vi "3x3 Smoothing.vi"(7 "Enable":bool, 11 "Image":u32[][](array[numeric])) -> (3 "Smoothed":u32[][](array[numeric]))   [LabVIEW 2017]
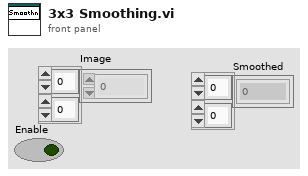
[diagram p1: front panel]
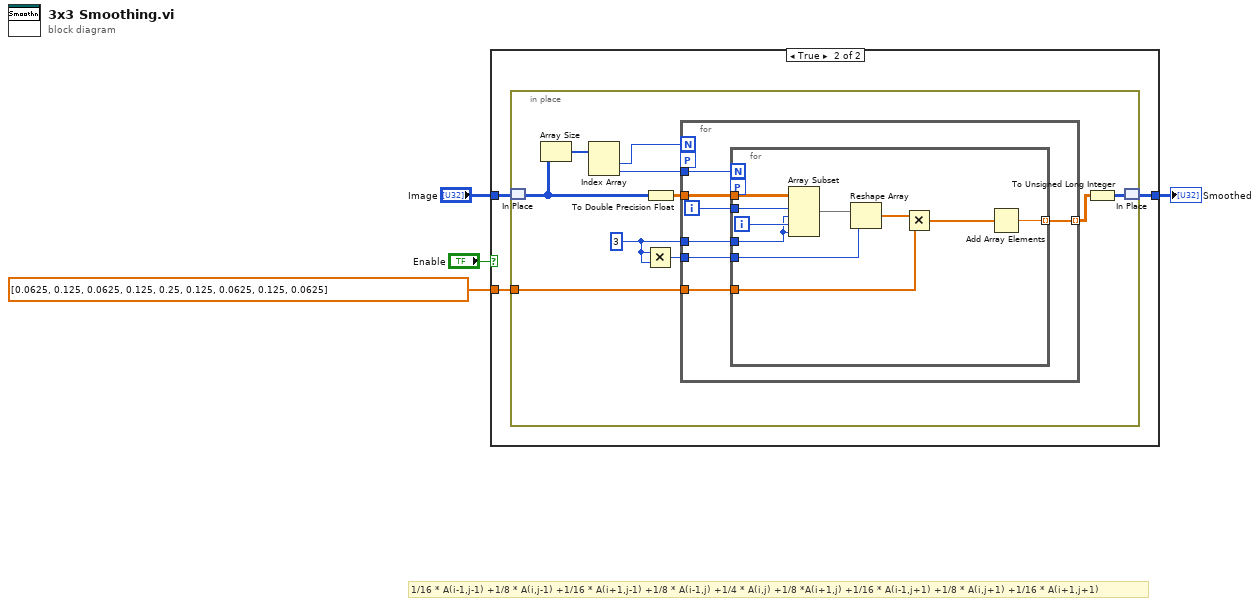
[diagram p0: block diagram]
diagram:
  # "1/16 * A(i-1,j-1) +1/8 * A(i,j-1) +1/16 * A(i+1,j-1) +1/8 * A(i-1,j) +1/4 * A(i,j) +1/8 *A(i+1,j) +1/16 * A(i-1,j+1) +1/8 * A(i,j+1) +1/16 * A(i+1,j+1)"
  n1 = case shown="True" "Enable" {
    tunnel: dbl[] [0.0625, 0.125, 0.0625, 0.125, 0.25, 0.125, 0.0625, 0.125, 0.0625] -> [_ w8]
    tunnel: "Image" -> [w5 w7]
    tunnel: [w5 w6] -> w2
    frame False {
    }
    frame True {
      n2 = in-place {
        in-place-border: w8 -> [w14]
        w12 = 3
        n3 = in-place-match #1(w7) -> (w10:u32[][])
        n4 = Array Size(array=w10) -> (size(s)=w18:i32[])
        n5 = Index Array(array=w18) -> (element #1=w15:i32, element #2=w17:i32)  [unwired: 2 in]
        n6 = Multiply(x=w12, y=w12) -> (x*y=w11:i32)
        n7 = To Double Precision Float(number=w10) -> (double precision float=w16:dbl[][])
        n8 = for {
          N: w15 -> [_]
          tunnel: w17 -> [w24]
          tunnel: w16 -> [w25]
          tunnel: w12 -> [w22]
          tunnel: w14 -> [w21]
          tunnel: [w20] -> w13 mode=indexing
          tunnel: w11 -> [w19]
          workers-P: _ -> [_]
          i -> [w23]
          n9 = for {
            N: w24 -> [_]
            tunnel: w25 -> [w35]
            tunnel: w23 -> [w34]
            tunnel: w22 -> [w32]
            tunnel: w21 -> [w30]
            tunnel: [w27] -> w20 mode=indexing
            tunnel: w19 -> [w26]
            workers-P: _ -> [_]
            i -> [w33]
            n10 = Array Subset(array=w35, index (row)=w34, length (row)=w32, index (col)=w33, length (col)=w32) -> (w31:dbl[][])
            n11 = Reshape Array(w31, w26) -> (w29:dbl[])
            n12 = Multiply(x=w29, y=w30) -> (x*y=w28:dbl[])
            n13 = Add Array Elements(numeric array=w28) -> (sum=w27:dbl)
          }
        }
        n14 = To Unsigned Long Integer(number=w13) -> (unsigned 32bit integer=w9:u32[][])
        n15 = in-place-match #1(w9) -> (w6:u32[][])
      }
    }
  }
  "Smoothed" <- w2
